vi "ScaleTo16Bit.vi"(8 "valid in":bool, 10 "factor":u16, 11 "Value in":fxp<+/-,32,14>) -> (0 "valid out":bool, 3 "16bit integer":i16)   [LabVIEW 2018]
uses:
  <vilib>/rvi/FXPMathLib/FxpConvert/subVIs/nifxpmath_Convert_SimConfig.ctl
  <vilib>/fxp/LVFixedPointQuantizationPolicyTypeDef.ctl
  <vilib>/fxp/LVFixedPointOverflowPolicyTypeDef.ctl
  <vilib>/rvi/FXPMathLib/FxpConvert/simVIs/DllFxpConvertTemp_sub.vi
  <vilib>/rvi/FXPMathLib/FxpConvert/XNode/nifxpmath_Convert.xnode
  <vilib>/rvi/FXPMathLib/FxpInterpret/XNode/nifxpmath_Interpret.xnode
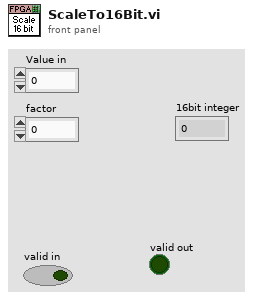
[diagram p1: front panel]
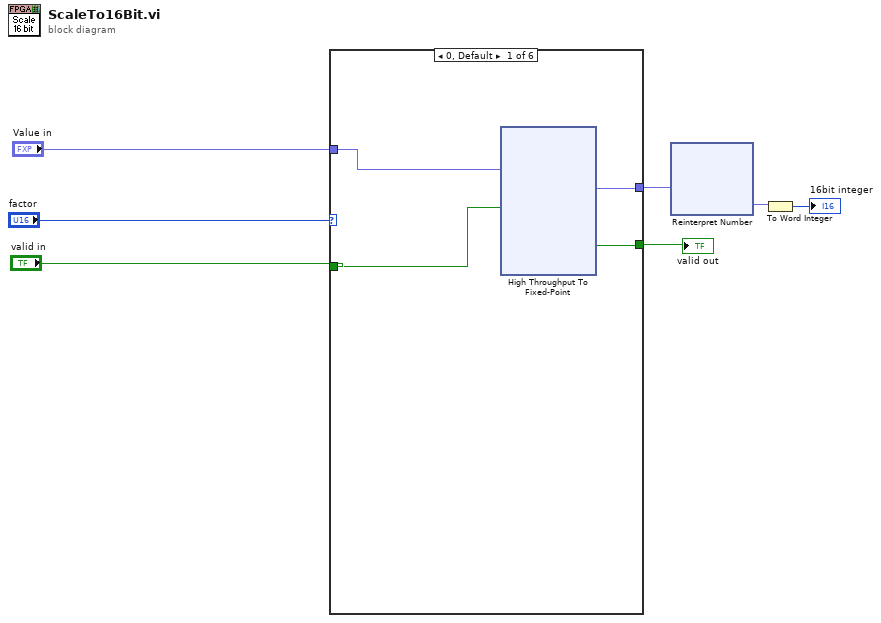
[diagram p0: block diagram]
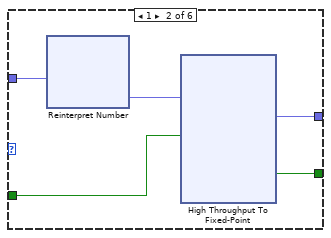
[diagram p2: hidden frame]
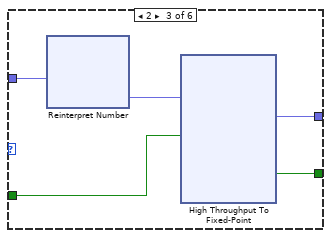
[diagram p3: hidden frame]
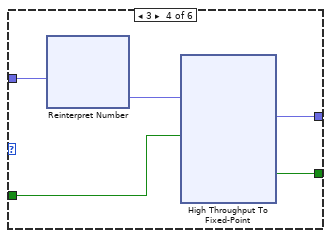
[diagram p4: hidden frame]
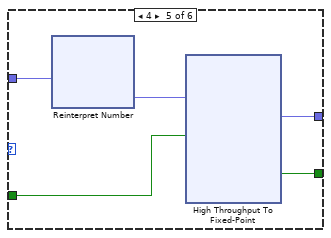
[diagram p5: hidden frame]
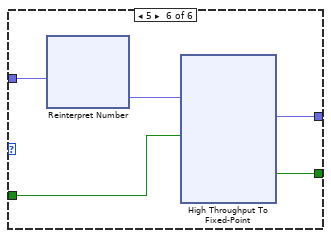
[diagram p6: hidden frame]
diagram:
  n1 = case shown="0, Default" "factor" {
    tunnel: "valid in" -> [w11 w38 w67 w96 w123 w154]
    tunnel: "Value in" -> [w8 w39 w68 w97 w126 w155]
    tunnel: [w9 w37 w65 w94 w124 w152] -> w4
    tunnel: [w10 w36 w66 w95 w125 w153] -> w3
    frame 0, Default {
      n2 = xnode "High Throughput To Fixed-Point"("x"=w8, "input valid"=w11) -> ("y"=w10:fxp<+/-,16,14>, "output valid"=w9:bool)  [unwired: 1 in, 1 out]
    }
    frame 1 {
      n3 = xnode "Reinterpret Number"("x"=w39) -> ("y"=w40:fxp<+/-,32,15>)
      n4 = xnode "High Throughput To Fixed-Point"("x"=w40, "input valid"=w38) -> ("y"=w36:fxp<+/-,16,14>, "output valid"=w37:bool)  [unwired: 1 in, 1 out]
    }
    frame 2 {
      n5 = xnode "Reinterpret Number"("x"=w68) -> ("y"=w69:fxp<+/-,32,16>)
      n6 = xnode "High Throughput To Fixed-Point"("x"=w69, "input valid"=w67) -> ("y"=w66:fxp<+/-,16,14>, "output valid"=w65:bool)  [unwired: 1 in, 1 out]
    }
    frame 3 {
      n7 = xnode "Reinterpret Number"("x"=w97) -> ("y"=w98:fxp<+/-,32,17>)
      n8 = xnode "High Throughput To Fixed-Point"("x"=w98, "input valid"=w96) -> ("y"=w95:fxp<+/-,16,14>, "output valid"=w94:bool)  [unwired: 1 in, 1 out]
    }
    frame 4 {
      n9 = xnode "Reinterpret Number"("x"=w126) -> ("y"=w127:fxp<+/-,32,18>)
      n10 = xnode "High Throughput To Fixed-Point"("x"=w127, "input valid"=w123) -> ("y"=w125:fxp<+/-,16,14>, "output valid"=w124:bool)  [unwired: 1 in, 1 out]
    }
    frame 5 {
      n11 = xnode "Reinterpret Number"("x"=w155) -> ("y"=w156:fxp<+/-,32,19>)
      n12 = xnode "High Throughput To Fixed-Point"("x"=w156, "input valid"=w154) -> ("y"=w153:fxp<+/-,16,14>, "output valid"=w152:bool)  [unwired: 1 in, 1 out]
    }
  }
  "valid out" <- w4
  n13 = xnode "Reinterpret Number"("x"=w3) -> ("y"=w2:fxp<+/-,16,16>)
  n14 = To Word Integer(number=w2) -> (16bit integer=→"16bit integer":i16)
